vi "Test20ISO+.vi"(8 "errin":errorcluster, 9 "L2T 2":T1 caption="Limites de test pris en compte", 10 "mesure":string, 11 "SN":string) -> (0 "error out":errorcluster, 3 "iso+":string)   [LabVIEW 2020]
uses:
  <vilib>/regexp/Match Regular Expression.xnode
  Ctrl/L2T.ctl
panel:
  # "Pre DCIR_____________________________________"
  # "intra DCIR_____________________________________"
  # "Post DCIR_____________________________________"
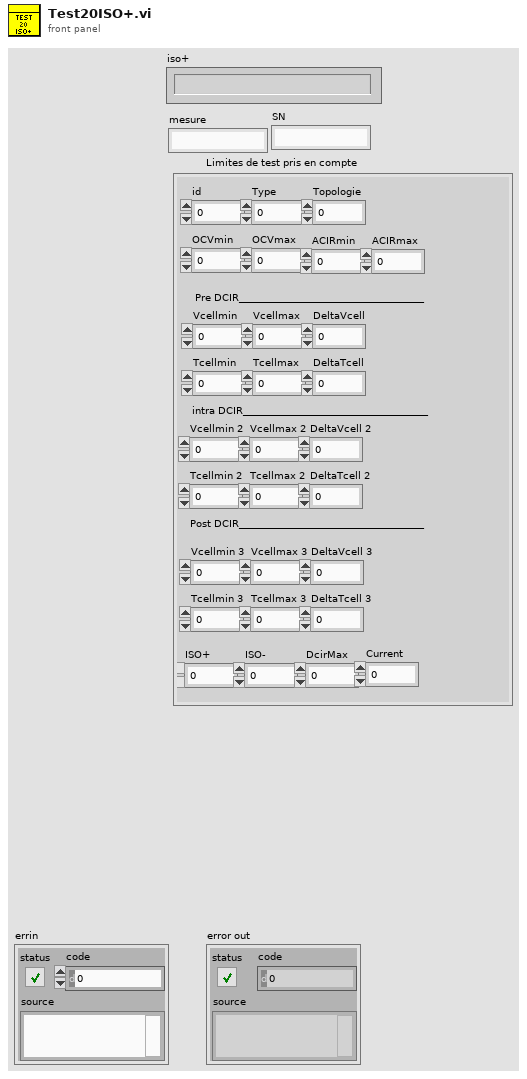
[diagram p1: front panel]
types:
  T1 = typedef "L2T.ctl" = cluster{"id":dbl, "Type":dbl, "OCVmin":dbl, "OCVmax":dbl, "ACIRmin":dbl, "ACIRmax":dbl, "Vcellmin":dbl, "Vcellmax":dbl, "DeltaVcell":dbl, "Tcellmin":dbl, "Tcellmax":dbl, "DeltaTcell":dbl, "ISO+":dbl, "ISO-":dbl, "DcirMax":dbl, "Current":dbl, "Topologie":dbl, "Vcellmin 2":dbl, "Vcellmax 2":dbl, "DeltaVcell 2":dbl, "Tcellmin 2":dbl, "Tcellmax 2":dbl, "DeltaTcell 2":dbl, "Vcellmin 3":dbl, "Vcellmax 3":dbl, "DeltaVcell 3":dbl, "Tcellmin 3":dbl, "Tcellmax 3":dbl, "DeltaTcell 3":dbl}
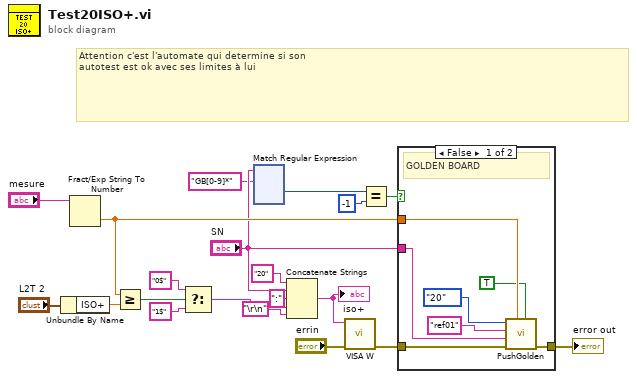
[diagram p0: block diagram]
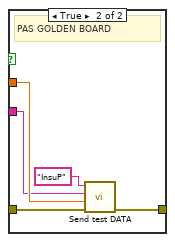
[diagram p2: hidden frame]
diagram:
  # "Attention c'est l'automate qui determine si son \nautotest est ok avec ses limites à lui"
  n1 = Unbundle By Name("L2T 2") -> ("ISO+"=w19:dbl)
  n2 = Fract/Exp String To Number(string="mesure") -> (number=w20:dbl)  [unwired: 3 in, 1 out]
  n3 = Greater Or Equal?(x=w20, y=w19) -> (x >= y?=w7:bool)
  n4 = Select(t="0$" ("chaîne"), s=w7, f="1$" ("chaîne")) -> (s? t:f=w10:string)
  n5 = xnode "Match Regular Expression"("input string"="SN", "regular expression"="GB[0-9]*") -> ("offset past match"=w13:i32)  [unwired: 4 in, 4 out]
  n6 = Concatenate Strings("20" ("chaîne"), "SN", ":" ("string"), w10, "\r\n") -> (w9:string)
  "iso+" <- w9
  n7 = call "VISA W.vi"("errin"="errin", "Chaîne"=w9) -> ("errout"=w2:errorcluster)  [unwired: 9 in]
  n8 = Equal?(x=w13, y=-1) -> (x = y?=w11:bool)
  n9 = case shown="False" w11 {
    tunnel: w20 -> [w23 w32]
    tunnel: [w27 w30] -> w18
    tunnel: "SN" -> [w25 w29]
    tunnel: w2 -> [w21 w28]
    frame False {
      # "GOLDEN BOARD"
      n10 = call "PushGolden.vi"("isInt?"=TRUE, "Value"=w23, "errin"=w21, "SN"=w25, "refFile"="ref01", "testnumber"=enum16{"50", "40", "30", "20", "11", "10", ""}."20") -> ("error out"=w27:errorcluster)  [unwired: 5 in]
    }
    frame True {
      # "PAS GOLDEN BOARD"
      n11 = call "Send test DATA.vi"("errin"=w28, "Value"=w32, "SN"=w29, "test"="InsuP") -> ("error out"=w30:errorcluster)  [unwired: 7 in]
    }
  }
  "error out" <- w18
